vi "Queue Comms FGV.vi"(7 "Action":T1, 8 "error in (no error)":errorcluster, 11 "queue In":refnum<queue>) -> (0 "error out":errorcluster, 3 "queue In":refnum<queue>)   [LabVIEW 2020, in "Error Handler.lvlib"]
uses:
  Error Handler.lvlib
  Queue FGV Action.ctl
  Private Controls/Element.ctl
  Private Controls/Module Action.ctl
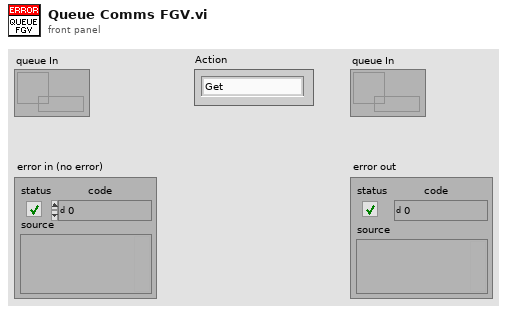
[diagram p1: front panel]
types:
  T1 = typedef "Error Handler.lvlib/Queue FGV Action.ctl" = enum16{"Get", "Set", "Release"}
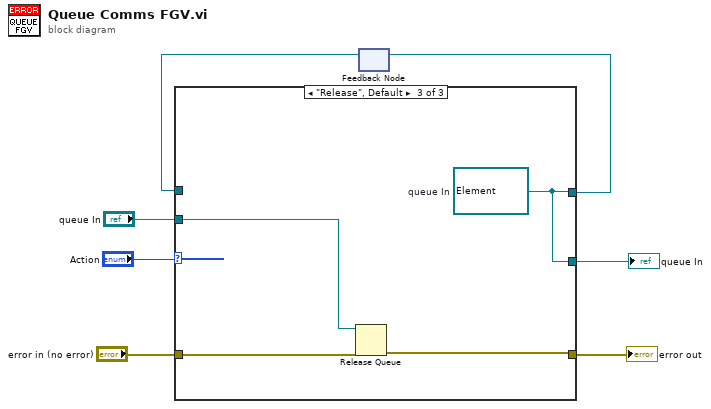
[diagram p0: block diagram]
diagram:
  n1 = feedback #1() -> (w3:refnum<queue>)  [unwired: 1 in]
  n2 = case shown="\"Release\", Default" "Action" {
    tunnel: "error in (no error)" -> [w9 w10 w15]
    tunnel: [w9 w10 w14] -> w5
    tunnel: "queue In" -> [_ w11 w13]
    tunnel: [w8 w11 w12] -> w4
    tunnel: [w8 w11 w12] -> w1
    tunnel: w3 -> [w8 _ _]
    frame "Get" {
    }
    frame "Set" {
    }
    frame "Release", Default {
      w12 = refnum<queue> refnum  # queue In
      n3 = Release Queue(queue=w13, error in (no error)=w15) -> (error out=w14:errorcluster)  [unwired: 1 in, 2 out]
    }
  }
  "error out" <- w5
  "queue In" <- w1
  n4 = feedback-in #1(w4) -> ()
